vi "TDOA Geometry VIs.vi"() -> ()   [LabVIEW 2025]
doc: "This example shows a Lissajous curve in an X/Y Graph. \n\nChoose the raw frequencies for X and Y and trim the movement with the Trim Slider.\n\nThis example uses the following Express VIs: Formula, Simulate Signal, and Build XY Graph."
uses:
  Instance           2 17Saved   Lissajous .vi
  <vilib>/express/express shared/transition.llb/Dynamic To Waveform Array.vi
  <vilib>/express/express arith-compare/Formula/Block/exnFormulaBlock how many pts in the wave.vi
  <vilib>/express/express shared/ex_Modify Signal Name.vi
  <vilib>/express/express shared/transition.llb/Waveform Array To Dynamic.vi
  <vilib>/express/express arith-compare/Formula/XNode/ExpressFormulaBlockNode.xnode
panel:
  in  "a":dbl(slide)=0.09048723897911828 scale=-1.0..1.0
  in  "f":i32(slide)=4 scale=0.0..10.0
  out "XY Graph":cluster{"Y":dbl[], "Y":dbl[]}[](graph)
  in  "Stop":bool
  # "Overview: Shows a TDOA equal time of arrival curve (hyperbola) based on \"a\" valiue (-1 to +1) in an XY Graph.\n(Eventually this will be a full blown TDOA simulation; right now the main purpose is merely to demonstrate LabView) \nInstructions:\n1. Run the VI.\n2. Choose the raw frequencies for X and Y.\n3. Trim the \"a\" value with the Trim slider.\n4. Click Stop to stop the VI."
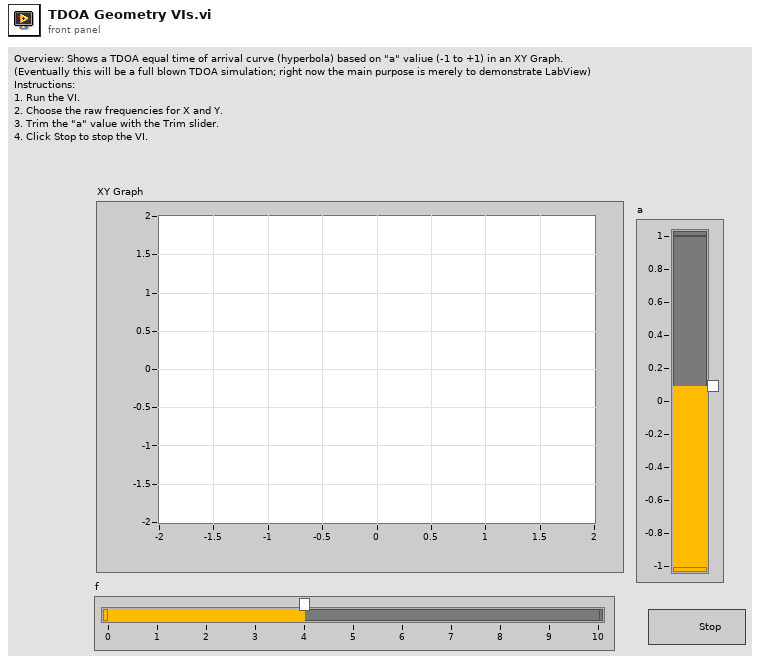
[diagram p1: front panel]
types:
  T1 = typedef "imagedata.ctl" = cluster{"image type":i32, "image depth":i32, "image":u8[], "mask":u8[], "colors":u32[], "Rectangle":cluster{"left":i16, "top":i16, "right":i16, "bottom":i16}}
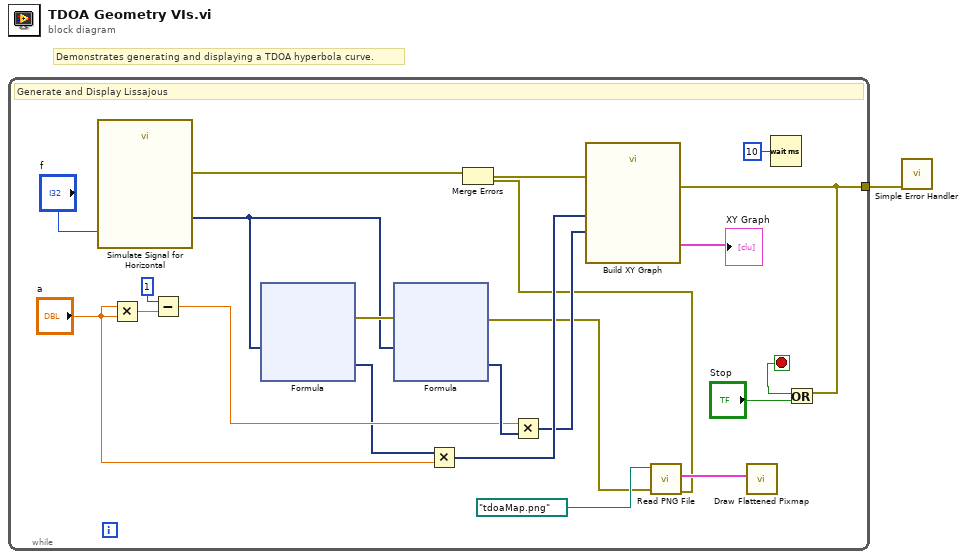
[diagram p0: block diagram]
diagram:
  # "Demonstrates generating and displaying a TDOA hyperbola curve."
  n1 = while {
    tunnel: [w17] -> w1
    stop <- w19 stop-if-true
    # "Generate and Display Lissajous"
    n2 = call "Simulate Signal for Horizontal"("Frequency"="f") -> ("Triangle"=w6:dynamicdata, "error out"=w20:errorcluster)  [unwired: 5 in, 8 out]
    n3 = Multiply(x="a", y="a") -> (x*y=w15:dbl)
    n4 = Subtract(x=u32 1 ("milliseconds to wait"), y=w15) -> (x-y=w12:dbl)
    n5 = xnode "Formula"("X"=w6) -> ("Result"=w10:dynamicdata, "error out"=w9:errorcluster)  [unwired: 1 in]
    n6 = xnode "Formula"("X"=w6, "error in (no error)"=w9) -> ("Result"=w13:dynamicdata, "error out"=w3:errorcluster)
    n7 = Multiply(x=w10, y="a") -> (x*y=w8:dynamicdata)
    n8 = Multiply(x=w12, y=w13) -> (x*y=w7:dynamicdata)
    n9 = call <vilib>:"Read PNG File.vi"("error in (no error)"=w3, "path to PNG file"=path "tdoaMap.png") -> ("error out"=w2:errorcluster, "image data"=w4:T1)  [unwired: 7 in, 1 out]
    n10 = Merge Errors(w20, w2) -> (w18:errorcluster)
    n11 = call "Build XY Graph"("error in (no error)"=w18, "Y Input"=w7, "X Input"=w8) -> ("error out"=w17:errorcluster, "XY Graph"=→"XY Graph":cluster{"Y":dbl[], "Y":dbl[]}[])  [unwired: 2 in, 5 out]
    n12 = call <vilib>:"Draw Flattened Pixmap.vi"("image data"=w4) -> ()  [unwired: 8 in, 1 out]
    n13 = Wait (ms)(milliseconds to wait=u32 10) -> ()  [unwired: 1 out]
    n14 = Or(x=w17, y="Stop") -> (x .or. y?=w19:bool)
  }
  n15 = call <vilib>:"Simple Error Handler.vi"("error in (no error)"=w1) -> ()  [unwired: 4 in, 5 out]
